vi "SDI-12 Single Operation with output cluster.vi"(0 "RS232 Port In":refnum<visa-resource-name>="COM11", 1 "Sensor Address In":string="0", 3 "Cumulative Volume":dbl, 4 "Sonde Data Ctl Refnum":refnum<vi>, 7 "Error In (No Error)":errorcluster, 8 "file directory (dialog if empty)":path=path "D:/Cascade/Raw Data files", 9 "Save File":bool, 12 "Time Array In":dbl[](array[numeric]), 13 "Measurement Array In":dbl[][](array[numeric])) -> (14 "time array out":dbl[](array[numeric]), 15 "Measurements Out":dbl[](array[numeric]), 16 "new file path (Not A Path if cancelled)":path, 17 "Time Array":timestamp[](array[timestamp]), 21 "Address Out":string="a" caption="sensor address out", 22 "Measurement  array Out":dbl[][](array[numeric]), 23 "output cluster":T1 caption="Cluster" {"Salinity" format="%_3g"; "Temp" format="%_2g"; "ORP" format="%_4g"; "pH" format="%_4g"; "Dissolved\nOxygen" format="%_3g"; "Specific\nConductance" format="%_4g"; "Cumulative\nVolume" format="%#_4g"}, 24 "Temperature":cluster{"Y":dbl[], "Y":dbl[]}[](graph), 25 "Sonde Data Display":T2, 27 "Error Out":errorcluster)   [LabVIEW 2016]
doc: "A general set of examples of the SDI-12 API for a generic sensor. A tab control separates each example, and contains the following examples:\n1. Read Single.\n2. Read Multiple.\n3. Acknowledge Active.\n4. Change Address.\n5. Address Query.\n6. Send Identification."
uses:
  SDI-12/Sonde Vertical Graph.ctl
  Waterloo DAQ/controls/Vertical Chart.ctl
  activeXtest/activeXtest 2015 Folder/sonde cluster.ctl
  <vilib>/Utility/file.llb/Write Delimited Spreadsheet (string).vi
  <vilib>/Utility/file.llb/Write Delimited Spreadsheet (DBL).vi
  SDI-12/SDI-12.lvlib
panel:
  out "loop counter":i32
  out "Error Out 3":errorcluster
  out "error out 2":errorcluster
  out "Error Out 2":errorcluster
  out "error out":errorcluster
  out "Sensor On/Off Response":bool
  out "Battery Voltage (V)":dbl
  out "Number of Measurements Out":i32
  in  "Measurement Type In (Normal)":i32(ring)=1 items=["Normal", "Concurrent", "Continuous"]
  out "Parameter Out":i32(ring) items=["0", "1", "2", "3", "4", "5", "6", "7", "8", "9"]
  in  "Parameter In (0)":i32(ring) items=["0", "1", "2", "3", "4", "5", "6", "7", "8", "9"]
  in  "CRC (False)":bool
  out "CRC Out":bool
  out "Measurement Type Out":i32(ring) items=["Normal", "Concurrent", "Continuous"]
  out "Time (s)":dbl
  out "start time":timestamp
  # "deg C"
  # "pH"
  # "specific conductance"
  # "salinity"
  # "DO % saturation"
  # "DO mg/L"
  # "ORP"
  # "depth"
  # "battery"
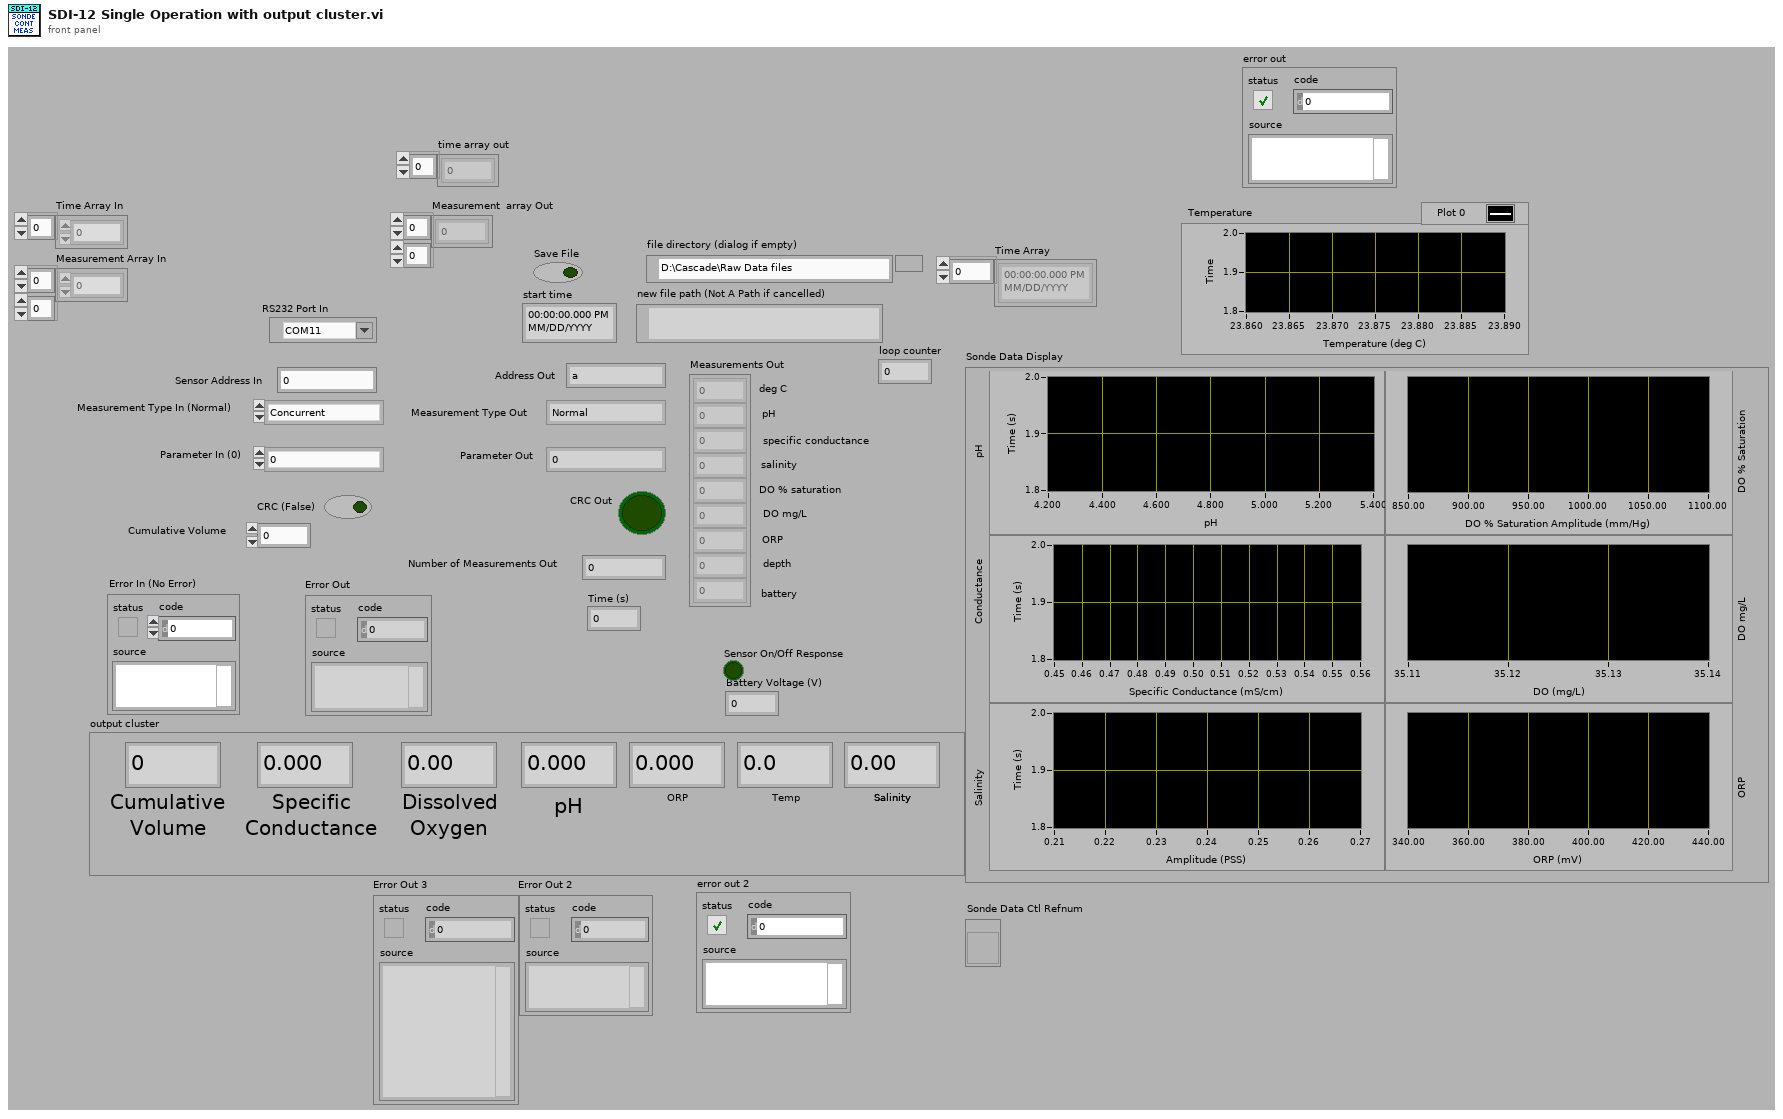
[diagram p1: front panel]
types:
  T1 = typedef "sonde cluster.ctl" = cluster{"Cumulative\nVolume":dbl, "Specific\nConductance":dbl, "Dissolved\nOxygen":dbl, "pH":dbl, "ORP":dbl, "Temp":dbl, "Salinity":dbl}
  T2 = typedef "Sonde Vertical Graph.ctl" = cluster{"pH":T3, "Conductance":T3, "Salinity":T3, "DO % Saturation":T3, "DO mg/L":T3, "ORP":T3}
  T3 = typedef "Vertical Chart.ctl" = cluster{"Y":dbl[], "Y":dbl[]}[]
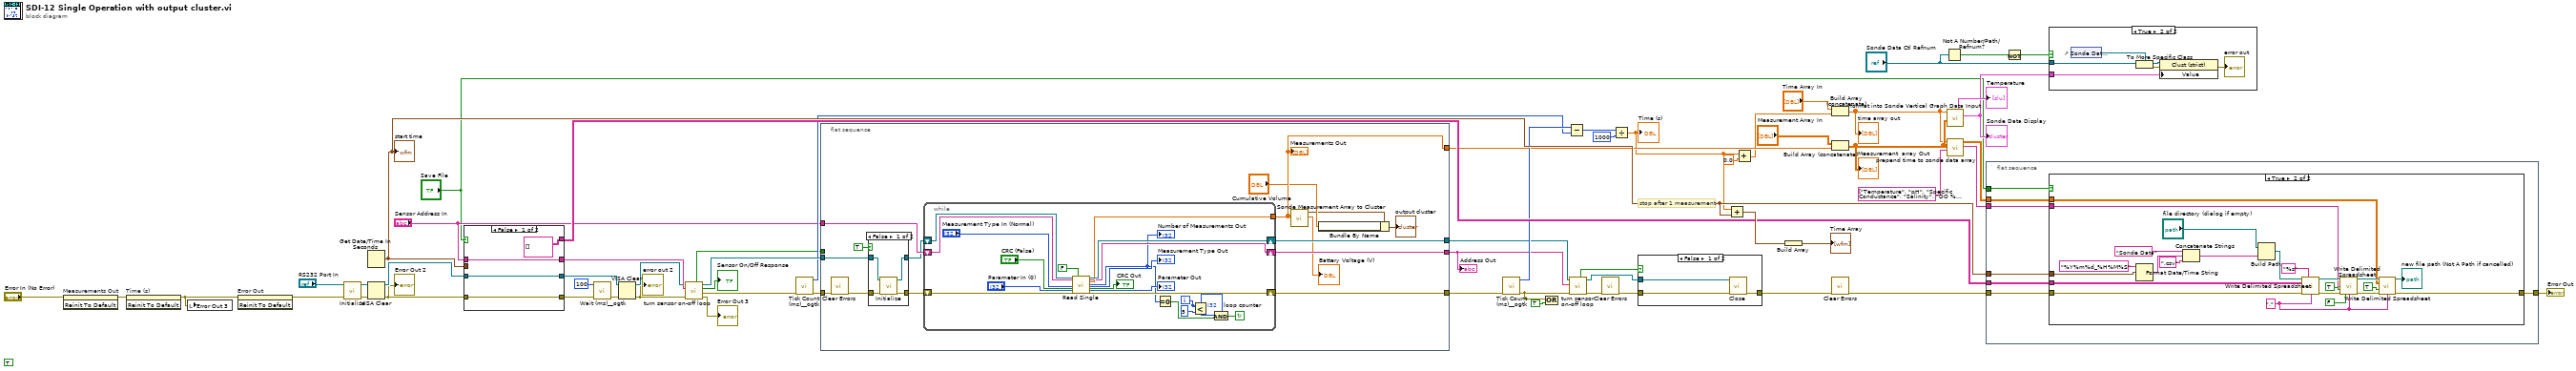
[diagram p0: block diagram]
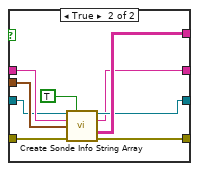
[diagram p2: hidden frame]
diagram:
  (unwired) TRUE ("Sensor On/Off")
  # "stop after 1 measurement"
  n1 = invoke on="Measurements Out" class="Arr (strict)" method="Reinit To Default"(error in="Error In (No Error)") -> (error out=w3:errorcluster)  [unwired: 2 in, 2 out]
  n2 = invoke on="Time (s)" class="DigNum (strict)" method="Reinit To Default"(error in=w3) -> (error out=w1:errorcluster)  [unwired: 2 in, 2 out]
  n3 = local write "Error Out 3"(w1) -> ()
  n4 = invoke on="Error Out" class="Clust (strict)" method="Reinit To Default"(error in=w1) -> (error out=w25:errorcluster)  [unwired: 2 in, 2 out]
  n5 = call "Initialize.vi"("Error In (No Error)"=w25, "RS232 Port In"="RS232 Port In") -> ("Error Out"=w16:errorcluster, "RS232 Port Out"=w59:refnum<visa-resource-name>)  [unwired: 8 in]
  n6 = Get Date/Time In Seconds() -> (seconds since 1Jan1904=w52:timestamp)
  "start time" <- w52
  n7 = VISA Clear(VISA resource name=w59, error in (no error)=w16) -> (VISA resource name out=w17:refnum<visa-resource-name>, error out=w15:errorcluster)
  "Error Out 2" <- w15
  n8 = case shown="False" "Save File" {
    tunnel: w52 -> [_ w73]
    tunnel: [string[][] [] ("Array") w72] -> w51
    tunnel: [w63 w71] -> w44
    tunnel: [w62 w70] -> w42
    tunnel: [w64 w69] -> w23
    tunnel: "Sensor Address In" -> [w62 w68]
    tunnel: w17 -> [w63 w67]
    tunnel: w15 -> [w64 w66]
    frame False {
    }
    frame True {
      n9 = call "Create Sonde Info String Array.vi"("VISA Refnum in"=w67, "Initialize/Close?"=TRUE, "Sensor Address In"=w68, "seconds since 1Jan1904"=w73, "error in (no error)"=w66) -> ("VISA Refnum out"=w71:refnum<visa-resource-name>, "Address Out"=w70:string, "Array"=w72:string[][], "error out"=w69:errorcluster)  [unwired: 7 in]
    }
  }
  n10 = call "Wait (ms)__ogtk.vi"("error in (no error)"=w23, "milliseconds to wait"=u32 100) -> ("error out"=w21:errorcluster)  [unwired: 8 in, 1 out]
  n11 = VISA Clear(VISA resource name=w44, error in (no error)=w21) -> (VISA resource name out=w24:refnum<visa-resource-name>, error out=w22:errorcluster)
  "error out 2" <- w22
  n12 = call "turn sensor on-off loop.vi"("error in (no error)"=w22, "Address Out"=w42, "VISA Refnum in"=w24) -> ("error out"=→"Error Out 3":errorcluster, "error out 2"=w45:errorcluster, "Sensor On/Off Response"=→"Sensor On/Off Response":bool, "VISA Refnum out"=w43:refnum<visa-resource-name>, "Initialize/Close?"=w14:bool)  [unwired: 4 in]
  n13 = call "Tick Count (ms)__ogtk.vi"("error in (no error)"=w45) -> ("error out"=w40:errorcluster, "millisecond timer value"=w38:u32)  [unwired: 9 in]
  n14 = flat-sequence {
    tunnel: [w88] -> w11
    tunnel: [w87] -> w41
    tunnel: w40 -> [w86]
    tunnel: w43 -> [w78]
    tunnel: [w84] -> w35
    tunnel: "Sensor Address In" -> [w85]
    tunnel: [w83] -> w8
    tunnel: w14 -> [_]
    frame #0 {
      n15 = call <vilib>:"Clear Errors.vi"("error in (no error)"=w86) -> ("error out"=w79:errorcluster)  [unwired: 5 in, 1 out]
      n16 = case shown="False" TRUE {
        tunnel: w79 -> [w112 w114]
        tunnel: w78 -> [w111 w113]
        tunnel: [w110 w114] -> w77
        tunnel: [w109 w113] -> w76
        frame False {
          n17 = call "Initialize.vi"("Error In (No Error)"=w112, "RS232 Port In"=w111) -> ("Error Out"=w110:errorcluster, "RS232 Port Out"=w109:refnum<visa-resource-name>)  [unwired: 8 in]
        }
        frame True {
        }
      }
      n18 = while {
        tunnel: [w99] -> w84
        shift-right: [w98] -> w83
        shift-left: w85 -> [w100]
        shift-right: [w107] -> w87
        shift-left: w77 -> [w97]
        shift-right: [w108] -> w88
        shift-left: w76 -> [w96]
        i -> [w91]
        stop <- w92 continue-if-true
        n19 = call "Read Single.vi"("RS232 Port In"=w96, "Sensor Address In"=w100, "Measurement Type In (Normal)"="Measurement Type In (Normal)", "CRC (False)"="CRC (False)", "Parameter In (0)"="Parameter In (0)", "Error In (No Error)"=w97, "Initialize/close"=FALSE) -> ("RS232 Port Out"=w108:refnum<visa-resource-name>, "Sensor Address Out"=w98:string, "Measurements Out"=w99:dbl[], "Number of Measurements Out"=w94:i32, "Measurement Type Out"=→"Measurement Type Out":i32, "CRC Out"=→"CRC Out":bool, "Parameter Out"=→"Parameter Out":i32, "Error Out"=w107:errorcluster)  [unwired: 13 in]
        "Number of Measurements Out" <- w94
        n20 = Equal To 0?(x=w94) -> (x = 0?=w93:bool)
        n21 = Less?(x=w91, y=5) -> (x < y?=w89:bool)
        n22 = And(x=w89, y=w93) -> (x .and. y?=w92:bool)
        "loop counter" <- w91
      }
      "Measurements Out" <- w84
      n23 = call "Sonde Measurement Array to Cluster.vi"("Measurements In"=w84) -> ("Battery Voltage (V)"=→"Battery Voltage (V)":dbl, "Sonde Data Cluster"=w81:T1)  [unwired: 9 in]
      n24 = Bundle By Name(cluster=w81, "Cumulative\nVolume"="Cumulative Volume") -> (→"output cluster":T1)
    }
  }
  n25 = call "Tick Count (ms)__ogtk.vi"("error in (no error)"=w41) -> ("error out"=w10:errorcluster, "millisecond timer value"=w39:u32)  [unwired: 9 in]
  n26 = Compound Arithmetic op=OR(w10, TRUE) -> ()  [unwired: 1 out]
  n27 = Subtract(x=w39, y=w38) -> (x-y=w37:u32)
  n28 = call "turn sensor on-off loop.vi"("error in (no error)"=w10, "Address Out"=w8, "VISA Refnum in"=w11) -> ("error out"=w7:errorcluster, "VISA Refnum out"=w9:refnum<visa-resource-name>, "Initialize/Close?"=w6:bool)  [unwired: 4 in, 2 out]
  n29 = call <vilib>:"Clear Errors.vi"("error in (no error)"=w7) -> ("error out"=w18:errorcluster)  [unwired: 5 in, 1 out]
  n30 = Divide(x=w37, y=u32 1000) -> (x/y=w34:dbl)
  "Time (s)" <- w34
  n31 = case shown="False" w6 {
    tunnel: [w117 w118] -> w55
    tunnel: w18 -> [w116 w118]
    tunnel: w9 -> [w115 _]
    frame False {
      n32 = call "Close.vi"("Error In (No Error)"=w116, "RS232 Port In"=w115) -> ("Error Out"=w117:errorcluster)  [unwired: 9 in]
    }
    frame True {
    }
  }
  n33 = Add(x=w34, y=w52) -> (x+y=w57:timestamp)
  n34 = Add(x=w34, y=0.0) -> (x+y=w33:dbl)
  n35 = Build Array(w57) -> (→"Time Array":timestamp[])
  n36 = Build Array (concatenate)("Time Array In", w33) -> (w48:dbl[])
  "time array out" <- w48
  n37 = Build Array (concatenate)("Measurement Array In", w35) -> (w56:dbl[][])
  "Measurement  array Out" <- w56
  n38 = call <vilib>:"Clear Errors.vi"("error in (no error)"=w55) -> ("error out"=w5:errorcluster)  [unwired: 5 in, 1 out]
  n39 = Not A Number/Path/Refnum?(number/path/refnum="Sonde Data Ctl Refnum") -> (NaN/Path/Refnum?=w31:bool)
  n40 = call "format into Sonde Vertical Graph Data Input.vi"("Sonde Measurement Array"=w56, "Time Array"=w48) -> ("Sonde Data Display"=w29:T2, "Temperature"=→"Temperature":cluster{"X":dbl[], "Y":dbl[]}[])  [unwired: 8 in]
  "Sonde Data Display" <- w29
  n41 = call "prepend time to sonde data array.vi"("Measurement Labels"=string[] ["Temperature", "pH", "Specific Conductance", "Salinity", "DO % saturation", "DO", "ORP", "depth", "battery"], "Sonde\nData Array"=w56, "Time Array"=w48) -> ("Header Array"=w50:string[], "Data Array"=w53:dbl[][])  [unwired: 7 in]
  n42 = flat-sequence {
    tunnel: w5 -> [w125]
    tunnel: [w124] -> w54
    tunnel: w50 -> [w123]
    tunnel: w53 -> [w122]
    tunnel: w52 -> [w121]
    tunnel: w51 -> [w120]
    tunnel: "Save File" -> [w119]
    frame #0 {
      n43 = case shown="True" w119 {
        tunnel: [w126 w146] -> w124
        tunnel: w125 -> [w126 w131]
        tunnel: w123 -> [_ w127]
        tunnel: w122 -> [_ w144]
        tunnel: w121 -> [_ w138]
        tunnel: w120 -> [_ w129]
        frame False {
        }
        frame True {
          w128 = "," ("delimiter (\\t)")
          n44 = Format Date/Time String(time format string (%c)="%Y%m%d_%H%M%S", seconds (now)=w138) -> (date/time string=w137:string)  [unwired: 1 in]
          n45 = Concatenate Strings("Sonde Data" ("name or relative path"), w137, ".csv" ("string")) -> (w139:string)
          n46 = Build Path(base path="file directory (dialog if empty)", name or relative path=w139) -> (appended path=w134:path)
          n47 = call-poly <vilib>:"Write Delimited Spreadsheet.vi"("file path (dialog if empty)"=w134, "format (%s)"="%s" ("format (%.3f)"), "2D data"=w129, "error in (no error)"=w131, "delimiter (\\t)"=w128) -> ("new file path (Not A Path if cancelled)"=w133:path, "error out"=w130:errorcluster)  [unwired: 9 in]
          n48 = call-poly <vilib>:"Write Delimited Spreadsheet.vi"("file path (dialog if empty)"=w133, "1D data"=w127, "append to file? (new file:F)"=TRUE ("append to file? (F)"), "error in (no error)"=w130, "transpose? (no:F)"=FALSE ("transpose? (F)"), "delimiter (\\t)"=w128) -> ("new file path (Not A Path if cancelled)"=w148:path, "error out"=w147:errorcluster)  [unwired: 8 in]
          n49 = call-poly <vilib>:"Write Delimited Spreadsheet.vi"("file path (dialog if empty)"=w148, "2D data"=w144, "append to file? (new file:F)"=TRUE ("append to file? (F)"), "error in (no error)"=w147, "delimiter (\\t)"=w128) -> ("new file path (Not A Path if cancelled)"=→"new file path (Not A Path if cancelled)":path, "error out"=w146:errorcluster)  [unwired: 9 in]
        }
      }
    }
  }
  n50 = Not(x=w31) -> (.not. x?=w30:bool)
  n51 = case shown="True" w30 {
    tunnel: w29 -> [_ w155]
    tunnel: "Sonde Data Ctl Refnum" -> [_ w153]
    frame False {
    }
    frame True {
      n52 = control-ref of="Sonde Data Display"() -> (w154:refnum<vi>)
      n53 = To More Specific Class(target class=w154, reference=w153) -> (specific class reference=w152:refnum<vi>, error out=w151:errorcluster)  [unwired: 1 in]
      n54 = property class="Clust (strict)"(reference=w152, error in=w151, "Value"=w155) -> (error out=→"error out":errorcluster)  [unwired: 1 out]
    }
  }
  "Error Out" <- w54
  "Address Out" <- w8
